vi "Laser349_RS232_Init.vi"(8 "error in (no error)":errorcluster, 9 "Laser ID Str":string, 10 "VISA resource name":refnum<visa-resource-name>, 11 "Laser349 in":refnum<class "Laser349.lvclass">) -> (0 "error out":errorcluster, 3 "Laser349 out":refnum<class "Laser349.lvclass">)   [LabVIEW 2018, in "Laser349.lvclass"]
uses:
  Laser349.lvclass
  Laser349.lvclass/Laser349.ctl
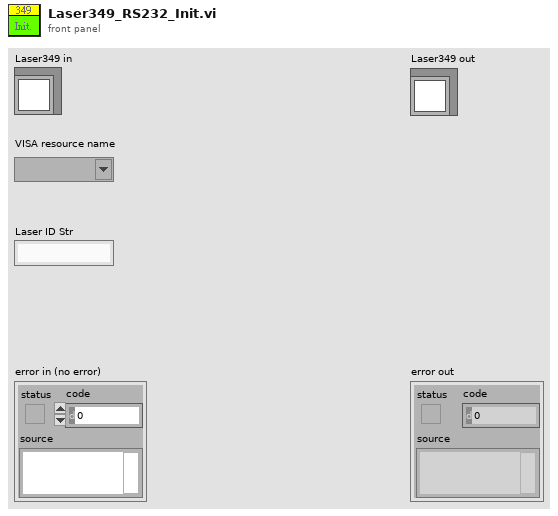
[diagram p1: front panel]
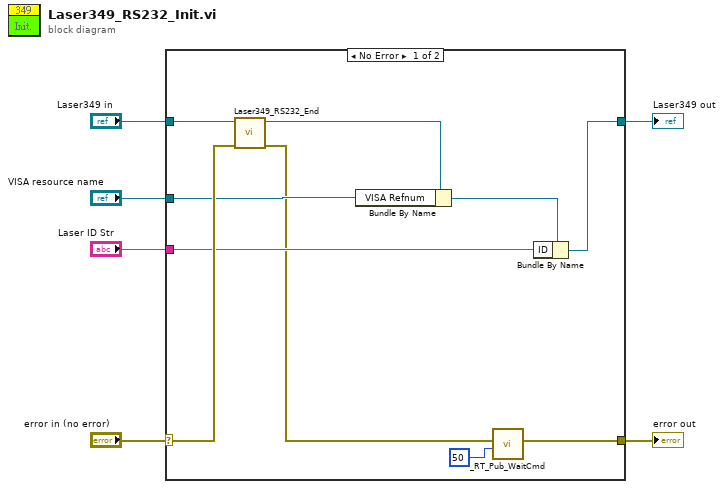
[diagram p0: block diagram]
diagram:
  n1 = case shown="No Error" "error in (no error)" {
    selector: "error in (no error)" -> [w14 w18]
    tunnel: [w7 w18] -> w5
    tunnel: [w15 w17] -> w4
    tunnel: "VISA resource name" -> [w13 _]
    tunnel: "Laser349 in" -> [w11 w17]
    tunnel: "Laser ID Str" -> [w12 _]
    frame No Error {
      n2 = call "Laser349_RS232_End.vi"("error in (no error)"=w14, "Laser349 in"=w11) -> ("error out"=w8:errorcluster, "Laser349 out"=w10:refnum<class "Laser349.lvclass">)  [unwired: 8 in]
      n3 = Bundle By Name(cluster=w10, "VISA Refnum"=w13) -> (w16:refnum<class "Laser349.lvclass">)
      n4 = call "_RT_Pub_WaitCmd.vi"("milliseconds to wait"=u32 50, "error in (no error)"=w8) -> ("error out"=w7:errorcluster)  [unwired: 9 in]
      n5 = Bundle By Name(cluster=w16, "ID"=w12) -> (w15:refnum<class "Laser349.lvclass">)
    }
    frame Error {
    }
  }
  "error out" <- w5
  "Laser349 out" <- w4
